vi "MAG_UI_Main.vi"() -> ()   [LabVIEW 2016]
doc: "Use this template to build a simple state machine design pattern. Each state executes code and determines which state to transition to."
uses:
  controls/MAG_UI_Data.ctl
  controls/MAG_UI_Command.ctl
  controls/MAG_Comms_State.ctl
  controls/Sensor_Data.ctl
  <vilib>/Math Plots/3D Math Plots/3D Surface/3D Surface XCtrl/3D Surface.xctl
  controls/MAG_UI_State.ctl
  controls/MAG_Display_State.ctl
  controls/MAG_UI_Comms_Config.ctl
  <vilib>/Math Plots/3D Math Plots/3D Surface/3D Surface Datatype/Public/Plot Helper (Matrix).vi
  <vilib>/Math Plots/3D Math Plots/3D Surface/3D Surface Datatype/3D Surface Datatype.lvclass
panel:
  in  "UI_Tab":enum32{"Display", "Config", "Debug"}(tab)
  out "Sensor Readings":dbl[][](array[numeric])=[[-533.0, -111.0, 239.0], [-402.0, 166.0, 184.0], [-184.0, 154.0, 29.0], [-106.0, 74.0, 11.0], [-532.0, -109.0, 246.0], [-398.0, 164.0, 175.0], [-205.0, 152.0, 32.0], [-119.0, 65.0, 9.0], [-529.0, -110.0, 242.0], [-408.0, 166.0, 184.0], [-198.0, 158.0, 27.0], [-108.0, 61.0, 6.0], [-539.0, -106.0, 240.0], [-407.0, 158.0, 183.0], [-191.0, 156.0, 28.0], [-113.0, 73.0, 15.0], [816.0, -260.0, 842.0], [539.0, 512.0, 512.0], [156.0, 425.0, 83.0], [13.0, 142.0, -72.0], [816.0, -262.0, 840.0], [528.0, 520.0, 512.0], [162.0, 425.0, 83.0], [13.0, 137.0, -84.0], [809.0, -260.0, 840.0], [538.0, 520.0, 504.0], [162.0, 432.0, 72.0], [13.0, 136.0, -84.0], [809.0, -260.0, 846.0], [538.0, 508.0, 512.0], [158.0, 435.0, 72.0], [19.0, 136.0, -79.0], [346.0, -168.0, 14.0], [287.0, -68.0, 19.0], [161.0, -34.0, 4.0], [70.0, -44.0, -7.0], [345.0, -191.0, 19.0], [279.0, -40.0, 8.0], [167.0, -16.0, 12.0], [72.0, -23.0, 2.0], [341.0, -190.0, 17.0], [285.0, -46.0, 9.0], [149.0, -15.0, 6.0], [54.0, -40.0, -2.0], [375.0, -201.0, 19.0], [282.0, -51.0, 10.0], [135.0, -37.0, 6.0], [81.0, -57.0, -12.0], [-80.0, -193.0, -48.0], [-73.0, -136.0, -12.0], [-5.0, -122.0, -31.0], [-19.0, -118.0, -17.0], [-118.0, -187.0, -48.0], [-73.0, -115.0, -22.0], [1.0, -113.0, -27.0], [-20.0, -111.0, -8.0], [-99.0, -184.0, -40.0], [-62.0, -145.0, -17.0], [0.0, -113.0, -37.0], [-7.0, -117.0, -15.0], [-126.0, -184.0, -50.0], [-72.0, -115.0, -14.0], [-4.0, -114.0, -25.0], [-29.0, -116.0, -14.0]]
  in  "Zero":bool=TRUE
  in  "Tab Control":enum32{"2D", "3D"}(tab)
  out "Node Response":T1(graph)
  in  "Node":i32
  out "3D Surface":refnum<class "3D Plot Datatype.lvclass">[](xcontrol)
  in  "Comms Setting":enum32{"Serial", "Bluetooth"}(tab)
  in  "VISA resource name":refnum<visa-resource-name>="COM11"
  in  "Serial Settings":T2={"baud rate"=115200, "data bits"=8, "parity"=enum."None", "stop bits"=10, "flow control"=0} {"flow control" items=["None"=0, "XON/XOFF"=1, "RTS/CTS"=2, "DTR/DSR"=4]; "stop bits" items=["1.0"=10, "1.5"=15, "2.0"=20]; "data bits" min=5 max=8 step=1; "baud rate" items=["75"=75, "110"=110, "134"=134, "150"=150, "300"=300, "600"=600, "1200"=1200, "1800"=1800, "2400"=2400, "4800"=4800, "7200"=7200, "9600"=9600, "14400"=14400, "19200"=19200, "28800"=28800, "38400"=38400, "56000"=56000, "57600"=57600, "115200"=115200, "128000"=128000, "230400"=230400]}
  out "Comm State":T3={"Comms_States"=enum."Send_Com", "Parameters"="", "Clear Buffer?"=FALSE}
  out "notification":T5
  out "comms":i32
  out "ui":i32
  in  "Button_Disconnect":bool
  in  "Button_Initialise":bool
  in  "Button_Stream":bool
  out "Status":T6
  in  "Button_Record":bool
  in  "Button_Sys_Check":bool
  in  "Button_Connect":bool
  in  "Button_Exit":bool
  # "MagBoard n64"
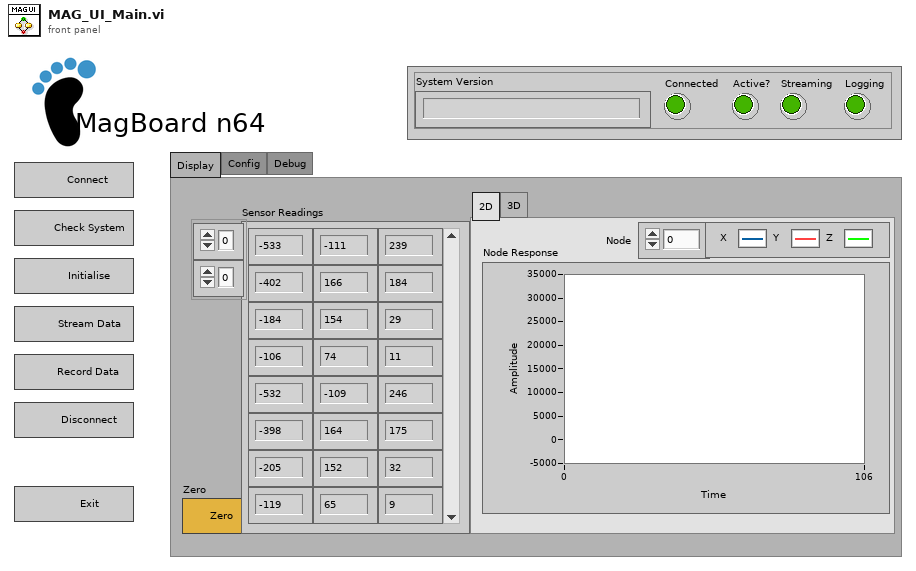
[diagram p1: front panel]
types:
  T1 = cluster{"Node XYZ List[0]":dbl, "Node XYZ List[1]":dbl, "Node XYZ List[2]":dbl}
  T2 = cluster{"baud rate":u32, "data bits":u16, "parity":enum16{"None", "Odd", "Even", "Mark", "Space"}, "stop bits":u16, "flow control":u16}
  T3 = typedef "MAG_UI_Command.ctl" = cluster{"Comms_States":T4, "Parameters":string, "Clear Buffer?":bool}
  T4 = typedef "MAG_Comms_State.ctl" = enum16{"Initialize", "Wait for Event", "Connect", "Send_Com", "Rcv_TXT", "Rcv_BIN", "Rcv_FILE", "Disconnect"}
  T5 = typedef "Sensor_Data.ctl" = cluster{"Time":u32, "Data":i16[]}
  T6 = typedef "MAG_UI_Data.ctl" = cluster{"System Version":string, "Connected":bool, "Active?":bool, "Streaming":bool, "Logging":bool}
  T7 = typedef "MAG_UI_Comms_Config.ctl" = cluster{enum16{"Serial", "Bluetooth"}, "Serial Refnum":refnum<visa-resource-name>}
  T8 = typedef "MAG_Display_State.ctl" = enum16{"Initialise", "Display", "Exit"}
  T9 = typedef "MAG_UI_State.ctl" = enum16{"Initialize", "Wait for Event", "Com_Connect", "Com_Init_Sys", "Com_Chk_Sys", "Com_Stream", "Com_Log", "Exit"}
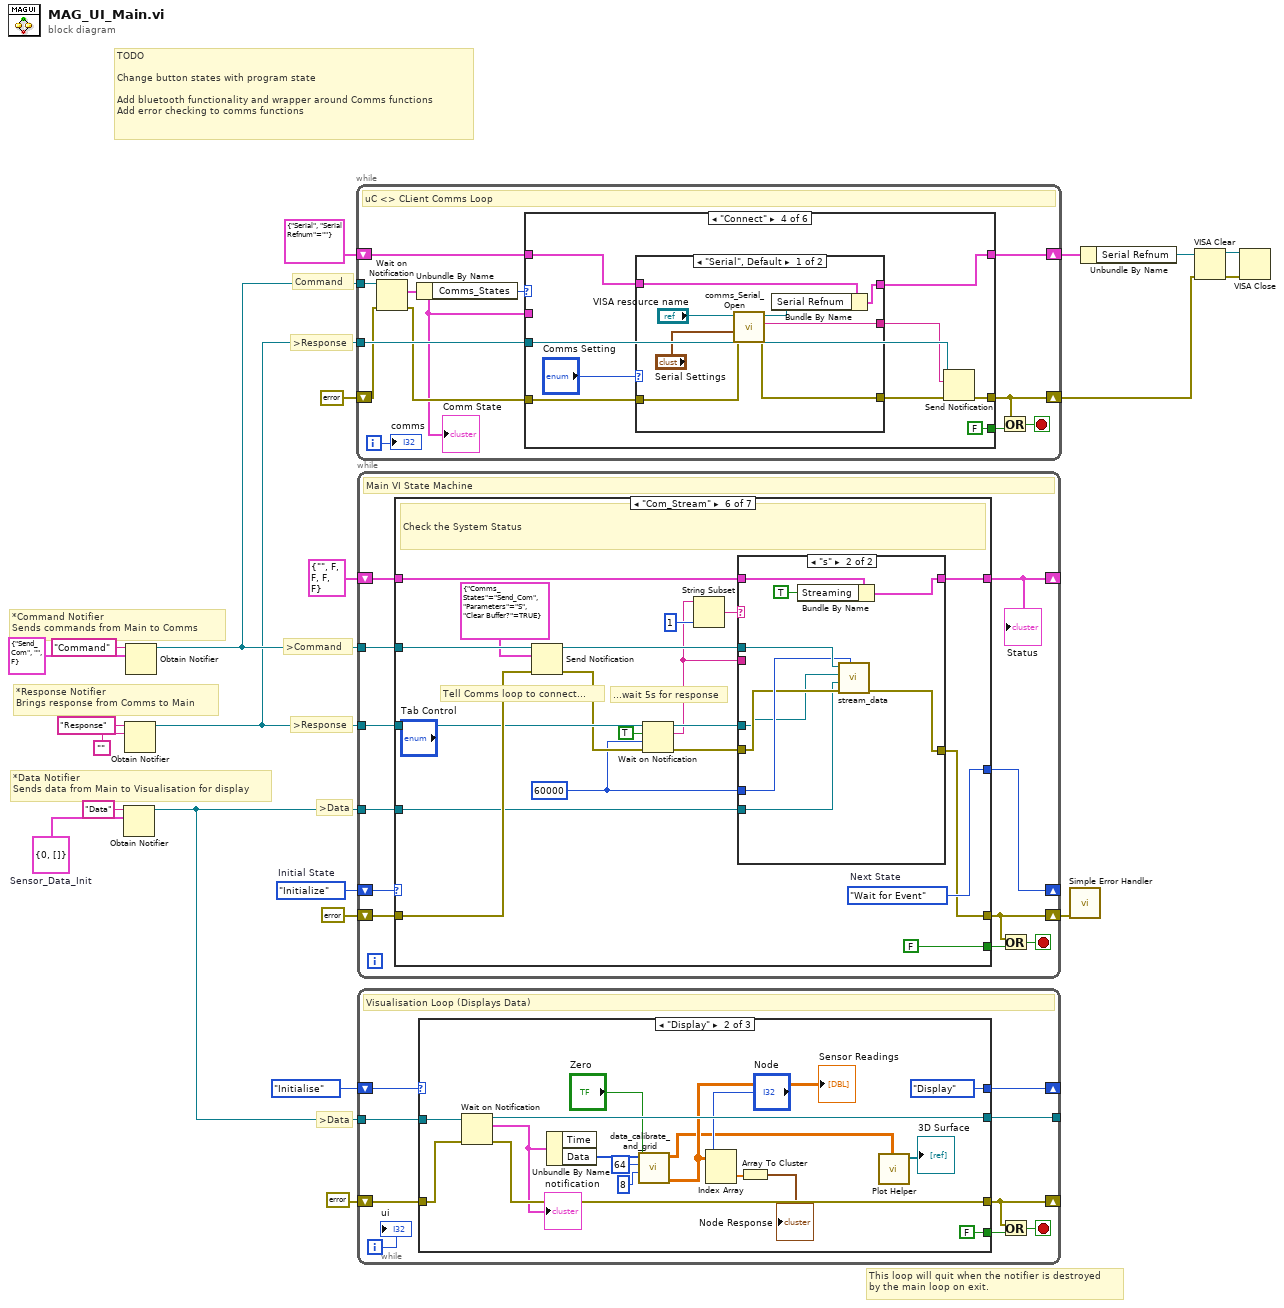
[diagram p0: block diagram]
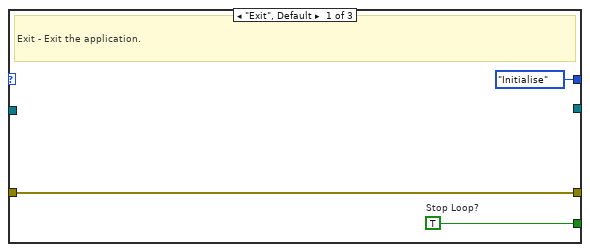
[diagram p2: hidden frame]
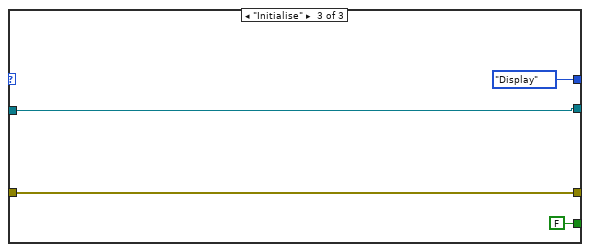
[diagram p3: hidden frame]
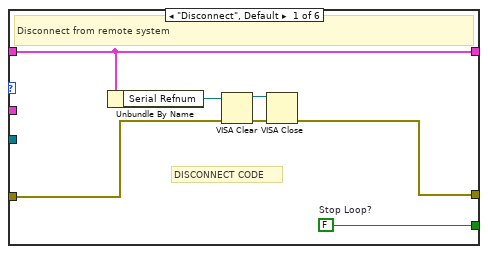
[diagram p4: hidden frame]
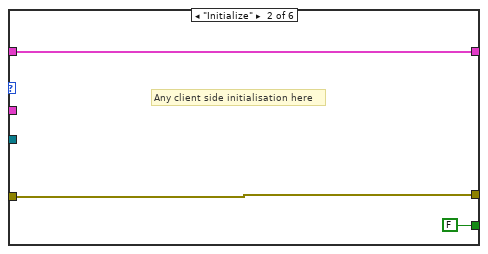
[diagram p5: hidden frame]
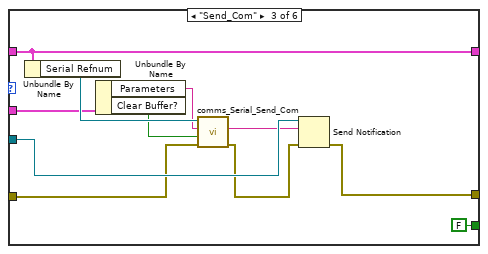
[diagram p6: hidden frame]
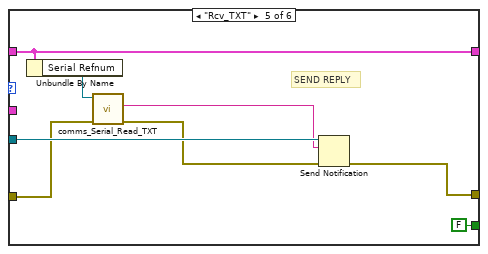
[diagram p8: hidden frame]
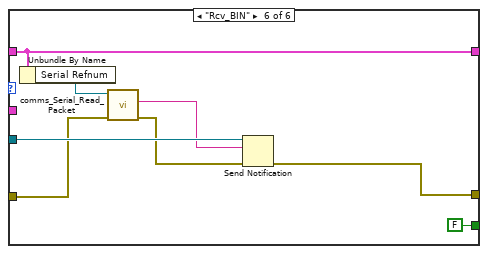
[diagram p9: hidden frame]
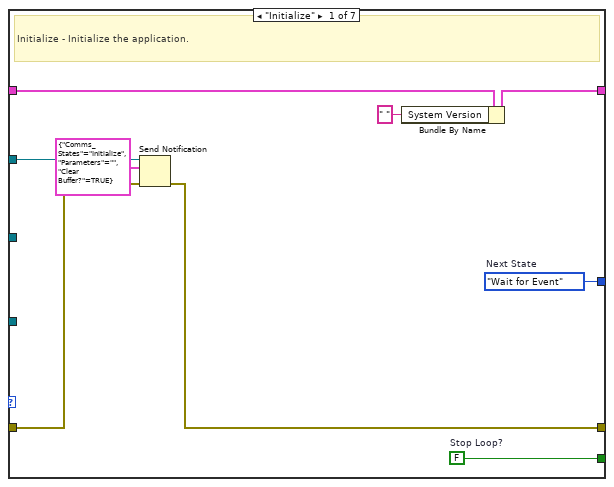
[diagram p10: hidden frame]
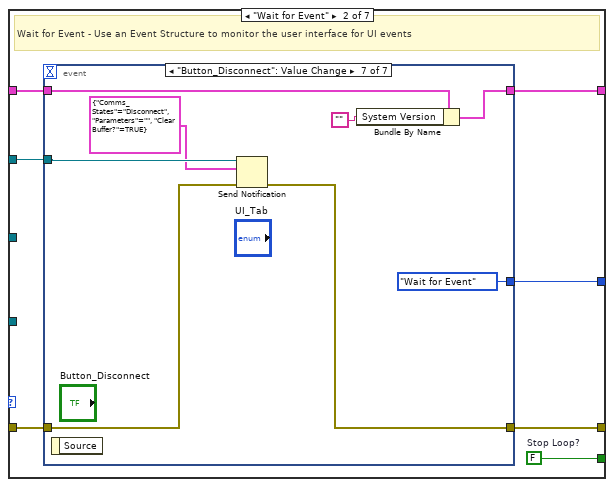
[diagram p11: hidden frame]
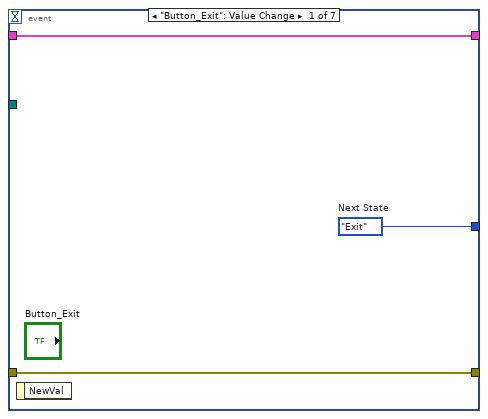
[diagram p12: hidden frame]
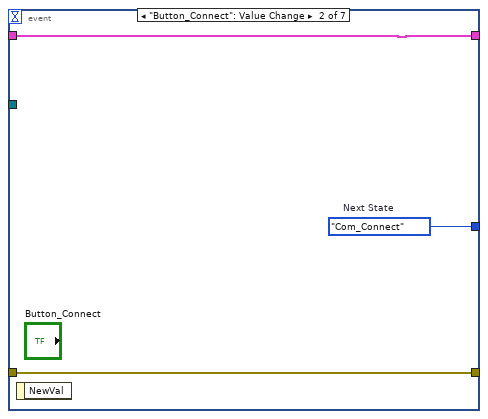
[diagram p13: hidden frame]
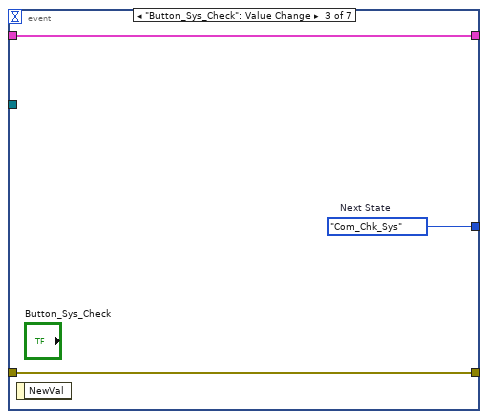
[diagram p14: hidden frame]
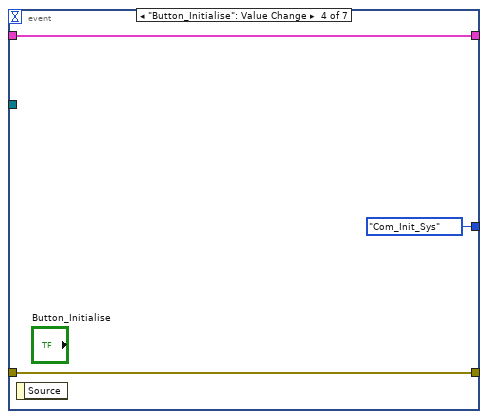
[diagram p15: hidden frame]
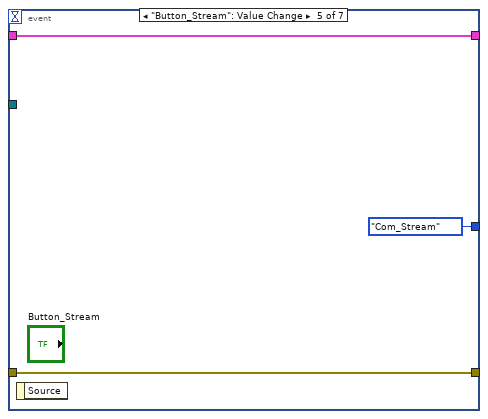
[diagram p16: hidden frame]
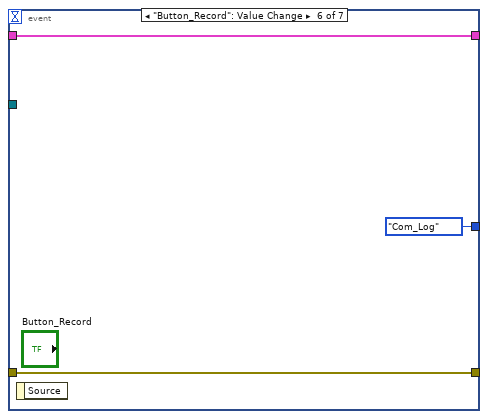
[diagram p17: hidden frame]
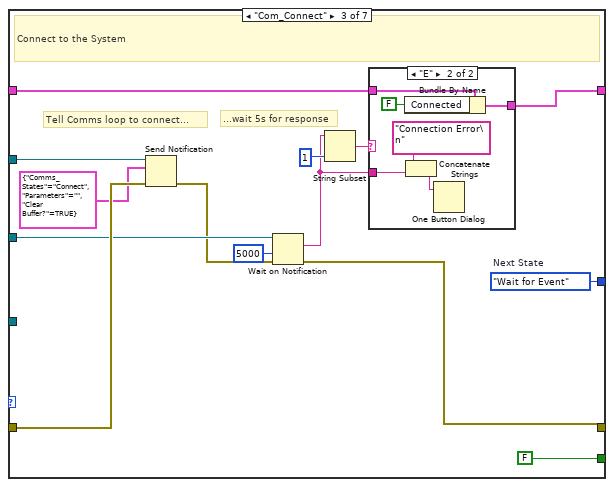
[diagram p18: hidden frame]
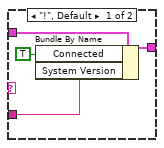
[diagram p19: hidden frame]
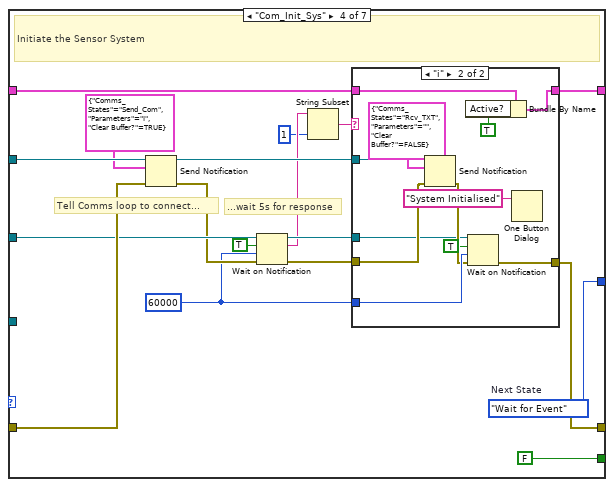
[diagram p20: hidden frame]
diagram:
  w10 = T5 {"Time"=0, "Data"=[]}  # Sensor_Data_Init
  w22 = MAG_UI_State."Initialize"  # Initial State
  # "TODO\n\nChange button states with program state\n\nAdd bluetooth functionality and wrapper around Comms functions\nAdd error checking to comms functions"
  # "This loop will quit when the notifier is destroyed\nby the main loop on exit."
  # ">Data"
  # ">Data"
  # ">Response"
  # ">Response"
  # ">Command"
  # "*Data Notifier\nSends data from Main to Visualisation for display"
  # "*Response Notifier\nBrings response from Comms to Main"
  # "*Command Notifier\nSends commands from Main to Comms"
  # "Command"
  n1 = Obtain Notifier(name (unnamed)="Data", notification data type=w10) -> (notifier out=w13:refnum<notifier>)  [unwired: 2 in, 2 out]
  n2 = Obtain Notifier(name (unnamed)="Response", notification data type="") -> (notifier out=w12:refnum<notifier>)  [unwired: 2 in, 2 out]
  n3 = Obtain Notifier(name (unnamed)="Command", notification data type=T3 {"Comms_States"=enum."Send_Com", "Parameters"="", "Clear Buffer?"=FALSE}) -> (notifier out=w16:refnum<notifier>)  [unwired: 2 in, 2 out]
  n4 = while {
    shift-right: [w31] -> w1
    shift-left: errorcluster {"status"=FALSE, "code"=0, "source"=""} ("error constant") -> [w28]
    tunnel: w16 -> [w30]
    tunnel: w12 -> [w32]
    shift-right: [w25] -> w2
    shift-left: T7 {enum."Serial", "Serial Refnum"=""} -> [w26]
    i -> [w24]
    stop <- w33 stop-if-true
    # "uC <> CLient Comms Loop"
    n5 = Wait on Notification(notifier=w30, error in (no error)=w28) -> (notification=w23:T3, error out=w27:errorcluster)  [unwired: 2 in, 2 out]
    "Comm State" <- w23
    n6 = Unbundle By Name(w23) -> ("Comms_States"=w29:T4)
    n7 = case shown="\"Connect\"" w29 {
      tunnel: [w41 FALSE ("Stop Loop?") FALSE ("Stop Loop?") FALSE ("Stop Loop?") FALSE ("Stop Loop?") FALSE ("Stop Loop?")] -> w34
      tunnel: w27 -> [w37 w43 w49 w57 w77 w84]
      tunnel: [w36 w43 w54 w64 w81 w89] -> w31
      tunnel: w32 -> [_ _ w55 w61 w82 w88]
      tunnel: w26 -> [w35 w42 w50 w59 w79 w85]
      tunnel: [w35 w42 w50 w58 w79 w85] -> w25
      tunnel: w23 -> [_ _ w46 _ _ _]
      frame "Disconnect", Default {
        w41 = FALSE  # Stop Loop?
        # "DISCONNECT CODE"
        # "Disconnect from remote system"
        n8 = Unbundle By Name(w35) -> ("Serial Refnum"=w40:refnum<visa-resource-name>)
        n9 = VISA Clear(VISA resource name=w40, error in (no error)=w37) -> (VISA resource name out=w38:refnum<visa-resource-name>, error out=w39:errorcluster)
        n10 = VISA Close(VISA resource name=w38, error in (no error)=w39) -> (error out=w36:errorcluster)
      }
      frame "Initialize" {
        # "Any client side initialisation here"
      }
      frame "Send_Com" {
        n11 = Unbundle By Name(w50) -> ("Serial Refnum"=w52:refnum<visa-resource-name>)
        n12 = Unbundle By Name(w46) -> ("Parameters"=w45:string, "Clear Buffer?"=w47:bool)
        n13 = call "comms_Serial_Send_Com.vi"("error in"=w49, "Buffer Clear?"=w47, "Command"=w45, "VISA resource in"=w52) -> ("error out"=w48:errorcluster, "Response"=w51:string)  [unwired: 5 in, 1 out]
        n14 = Send Notification(notification=w51, notifier=w55, error in (no error)=w48) -> (error out=w54:errorcluster)  [unwired: 1 out]
      }
      frame "Connect" {
        n15 = case shown="\"Serial\", Default" "Comms Setting" {
          tunnel: [w66 w73] -> w60
          tunnel: w59 -> [w70 w74]
          tunnel: [w68 w74] -> w58
          tunnel: w57 -> [w67 w73]
          tunnel: [w65 _] -> w56
          frame "Serial", Default {
            n16 = call "comms_Serial_Open.vi"("error in (no error)"=w67, "Serial Settings in"="Serial Settings", "VISA Refnum in"="VISA resource name") -> ("error out"=w66:errorcluster, "Data Out"=w65:string, "VISA Refnum out"=w69:refnum<visa-resource-name>)  [unwired: 6 in]
            n17 = Bundle By Name(cluster=w70, "Serial Refnum"=w69) -> (w68:T7)
          }
          frame "Bluetooth" {
          }
        }
        n18 = Send Notification(notification=w56, notifier=w61, error in (no error)=w60) -> (error out=w64:errorcluster)  [unwired: 1 out]
      }
      frame "Rcv_TXT" {
        # "SEND REPLY"
        n19 = Unbundle By Name(w79) -> ("Serial Refnum"=w78:refnum<visa-resource-name>)
        n20 = call "comms_Serial_Read_TXT.vi"("error in"=w77, "VISA resource in"=w78) -> ("error out"=w76:errorcluster, "Data Out"=w75:string)  [unwired: 6 in, 2 out]
        n21 = Send Notification(notification=w75, notifier=w82, error in (no error)=w76) -> (error out=w81:errorcluster)  [unwired: 1 out]
      }
      frame "Rcv_BIN" {
        n22 = Unbundle By Name(w85) -> ("Serial Refnum"=w86:refnum<visa-resource-name>)
        n23 = call "comms_Serial_Read_Packet.vi"("error in"=w84, "VISA resource in"=w86) -> ("error out"=w83:errorcluster, "Data Out"=w87:string)  [unwired: 7 in, 1 out]
        n24 = Send Notification(notification=w87, notifier=w88, error in (no error)=w83) -> (error out=w89:errorcluster)  [unwired: 1 out]
      }
    }
    n25 = Or(x=w31, y=w34) -> (x .or. y?=w33:bool)
    "comms" <- w24
  }
  n26 = while {
    shift-right: [w100] -> _
    shift-left: w22 -> [w101]
    shift-right: [w91] -> _
    shift-left: T6 {"System Version"="", "Connected"=FALSE, "Active?"=FALSE, "Streaming"=FALSE, "Logging"=FALSE} ("Data") -> [w99]
    shift-right: [w95] -> w19
    shift-left: errorcluster {"status"=FALSE, "code"=0, "source"=""} ("error constant") -> [w98]
    tunnel: w16 -> [w94]
    tunnel: w12 -> [w93]
    tunnel: w13 -> [w92]
    stop <- w96 stop-if-true
    # "Main VI State Machine"
    n27 = case shown="\"Com_Stream\"" w101 {
      tunnel: [w110 w117 w157 w176 w213 w249 w285] -> w100
      tunnel: [w109 w116 FALSE ("Stop Loop?") FALSE ("Stop Loop?") FALSE ("Stop Loop?") FALSE ("Stop Loop?") w283] -> w97
      tunnel: w99 -> [w108 w115 w149 w180 w217 w253 w284]
      tunnel: [w107 w114 w148 w179 w216 w252 w284] -> w91
      tunnel: w98 -> [w103 w113 w154 w183 w220 w256 w279]
      tunnel: [w102 w112 w151 w173 w210 w246 w278] -> w95
      tunnel: w94 -> [w105 w111 w155 w184 w221 w257 w282]
      tunnel: w93 -> [_ _ w153 w182 w219 w255 w276]
      tunnel: w92 -> [_ _ _ _ _ w242 w275]
      frame "Initialize" {
        w109 = FALSE  # Stop Loop?
        w110 = MAG_UI_State."Wait for Event"  # Next State
        # "Initialize - Initialize the application."
        n28 = Send Notification(notification=T3 {"Comms_States"=enum."Initialize", "Parameters"="", "Clear Buffer?"=TRUE}, notifier=w105, error in (no error)=w103) -> (error out=w102:errorcluster)  [unwired: 1 out]
        n29 = Bundle By Name(cluster=w108, "System Version"=" ") -> (w107:T6)
      }
      frame "Wait for Event" {
        w116 = FALSE  # Stop Loop?
        # "Wait for Event - Use an Event Structure to monitor the user interface for UI events"
        n30 = event shown="[6] \"Button_Disconnect\": Value Change" {
          selector: _ -> [_ _ _ _ _ _ _]
          dyn-events: _ -> [_ _ _ _ _ _ _]
          timeout: _ -> [_ _ _ _ _ _ _]
          tunnel: [w120 w123 w126 MAG_UI_State."Com_Init_Sys" ("Next State") MAG_UI_State."Com_Stream" ("Next State") MAG_UI_State."Com_Log" ("Next State") MAG_UI_State."Wait for Event" ("Next State")] -> w117
          tunnel: w115 -> [w119 w121 w124 w129 w132 w135 w138]
          tunnel: [w119 w121 w124 w129 w132 w135 w137] -> w114
          tunnel: w113 -> [w118 w122 w125 w128 w131 w134 w141]
          tunnel: [w118 w122 w125 w128 w131 w134 w140] -> w112
          tunnel: w111 -> [_ _ _ _ _ _ w142]
          event "Button_Exit": Value Change {
            w120 = MAG_UI_State."Exit"  # Next State
            n31 = event-data() -> ()  [unwired: 1 in, 1 out]
          }
          event "Button_Connect": Value Change {
            w123 = MAG_UI_State."Com_Connect"  # Next State
            n32 = event-data() -> ()  [unwired: 1 in, 1 out]
          }
          event "Button_Sys_Check": Value Change {
            w126 = MAG_UI_State."Com_Chk_Sys"  # Next State
            n33 = event-data() -> ()  [unwired: 1 in, 1 out]
          }
          event "Button_Initialise": Value Change {
            n34 = event-data() -> ()  [unwired: 1 in, 1 out]
          }
          event "Button_Stream": Value Change {
            n35 = event-data() -> ()  [unwired: 1 in, 1 out]
          }
          event "Button_Record": Value Change {
            n36 = event-data() -> ()  [unwired: 1 in, 1 out]
          }
          event "Button_Disconnect": Value Change {
            n37 = event-data() -> ()  [unwired: 1 in, 1 out]
            n38 = Send Notification(notification=T3 {"Comms_States"=enum."Disconnect", "Parameters"="", "Clear Buffer?"=TRUE}, notifier=w142, error in (no error)=w141) -> (error out=w140:errorcluster)  [unwired: 1 out]
            n39 = Bundle By Name(cluster=w138, "System Version"="") -> (w137:T6)
          }
        }
      }
      frame "Com_Connect" {
        w157 = MAG_UI_State."Wait for Event"  # Next State
        # "...wait 5s for response"
        # "Tell Comms loop to connect..."
        # "Connect to the System"
        n40 = Send Notification(notification=T3 {"Comms_States"=enum."Connect", "Parameters"="", "Clear Buffer?"=TRUE}, notifier=w155, error in (no error)=w154) -> (error out=w152:errorcluster)  [unwired: 1 out]
        n41 = Wait on Notification(notifier=w153, timeout in ms (-1)=5000, error in (no error)=w152) -> (notification=w144:string, error out=w151:errorcluster)  [unwired: 1 in, 2 out]
        n42 = String Subset(string=w144, length (rest)=1 ("offset (0)")) -> (substring=w146:string)  [unwired: 1 in]
        n43 = case shown="\"E\"" w146 {
          tunnel: w149 -> [w161 w165]
          tunnel: [w160 w164] -> w148
          tunnel: w144 -> [w158 w162]
          frame "!", Default {
            n44 = Bundle By Name(cluster=w161, "Connected"=TRUE, "System Version"=w158) -> (w160:T6)
          }
          frame "E" {
            n45 = Bundle By Name(cluster=w165, "Connected"=FALSE) -> (w164:T6)
            n46 = Concatenate Strings("Connection Error\n", w162) -> (w167:string)
            n47 = One Button Dialog(message=w167) -> ()  [unwired: 1 in, 1 out]
          }
        }
      }
      frame "Com_Init_Sys" {
        w176 = MAG_UI_State."Wait for Event"  # Next State
        w175 = 60000 ("timeout in ms (-1)")
        # "...wait 5s for response"
        # "Tell Comms loop to connect..."
        # "Initiate the Sensor System"
        n48 = Send Notification(notification=T3 {"Comms_States"=enum."Send_Com", "Parameters"="I", "Clear Buffer?"=TRUE}, notifier=w184, error in (no error)=w183) -> (notifier out=w177:refnum<notifier>, error out=w181:errorcluster)
        n49 = Wait on Notification(notifier=w182, ignore previous (F)=TRUE, timeout in ms (-1)=w175, error in (no error)=w181) -> (notifier out=w172:refnum<notifier>, notification=w169:string, error out=w174:errorcluster)  [unwired: 1 out]
        n50 = String Subset(string=w169, length (rest)=1 ("offset (0)")) -> (substring=w170:string)  [unwired: 1 in]
        n51 = case shown="\"i\"" w170 {
          selector: w170 -> [w190 _]
          tunnel: w180 -> [w189 w196]
          tunnel: [w188 w195] -> w179
          tunnel: w177 -> [_ w203]
          tunnel: w175 -> [_ w202]
          tunnel: w174 -> [w186 w201]
          tunnel: [w186 w199] -> w173
          tunnel: w172 -> [_ w198]
          frame "E", Default {
            n52 = Bundle By Name(cluster=w189, "Connected"=FALSE) -> (w188:T6)
            n53 = Concatenate Strings("Initialisation Failed", w190) -> (w192:string)
            n54 = One Button Dialog(message=w192) -> ()  [unwired: 1 in, 1 out]
          }
          frame "i" {
            n55 = Send Notification(notification=T3 {"Comms_States"=enum."Rcv_TXT", "Parameters"="", "Clear Buffer?"=FALSE}, notifier=w203, error in (no error)=w201) -> (error out=w200:errorcluster)  [unwired: 1 out]
            n56 = Bundle By Name(cluster=w196, "Active?"=TRUE) -> (w195:T6)
            n57 = Wait on Notification(notifier=w198, ignore previous (F)=TRUE, timeout in ms (-1)=w202, error in (no error)=w200) -> (error out=w199:errorcluster)  [unwired: 3 out]
            n58 = One Button Dialog(message="System Initialised") -> ()  [unwired: 1 in, 1 out]
          }
        }
      }
      frame "Com_Chk_Sys" {
        w213 = MAG_UI_State."Wait for Event"  # Next State
        w212 = 5000 ("timeout in ms (-1)")
        # "...wait 5s for response"
        # "Tell Comms loop to connect..."
        # "Check the System Status"
        n59 = Send Notification(notification=T3 {"Comms_States"=enum."Send_Com", "Parameters"="C", "Clear Buffer?"=TRUE}, notifier=w221, error in (no error)=w220) -> (notifier out=w214:refnum<notifier>, error out=w218:errorcluster)
        n60 = Wait on Notification(notifier=w219, ignore previous (F)=TRUE, timeout in ms (-1)=w212, error in (no error)=w218) -> (notifier out=w209:refnum<notifier>, notification=w206:string, error out=w211:errorcluster)  [unwired: 1 out]
        n61 = String Subset(string=w206, length (rest)=1 ("offset (0)")) -> (substring=w207:string)  [unwired: 1 in]
        n62 = case shown="\"c\"" w207 {
          selector: w207 -> [w227 _]
          tunnel: w217 -> [w226 w239]
          tunnel: [w225 w239] -> w216
          tunnel: w214 -> [_ w237]
          tunnel: w212 -> [_ w236]
          tunnel: w211 -> [w223 w235]
          tunnel: [w223 w233] -> w210
          tunnel: w209 -> [_ w232]
          frame "E", Default {
            n63 = Bundle By Name(cluster=w226, "Connected"=FALSE) -> (w225:T6)
            n64 = Concatenate Strings("Initialisation Failed", w227) -> (w229:string)
            n65 = One Button Dialog(message=w229) -> ()  [unwired: 1 in, 1 out]
          }
          frame "c" {
            n66 = Send Notification(notification=T3 {"Comms_States"=enum."Rcv_TXT", "Parameters"="", "Clear Buffer?"=FALSE}, notifier=w237, error in (no error)=w235) -> (error out=w234:errorcluster)  [unwired: 1 out]
            n67 = Wait on Notification(notifier=w232, ignore previous (F)=TRUE, timeout in ms (-1)=w236, error in (no error)=w234) -> (notification=w231:string, error out=w233:errorcluster)  [unwired: 2 out]
            n68 = One Button Dialog(message=w231) -> ()  [unwired: 1 in, 1 out]
          }
        }
      }
      frame "Com_Stream" {
        w249 = MAG_UI_State."Wait for Event"  # Next State
        w248 = 60000 ("timeout in ms (-1)")
        # "...wait 5s for response"
        # "Tell Comms loop to connect..."
        # "Check the System Status"
        n69 = Send Notification(notification=T3 {"Comms_States"=enum."Send_Com", "Parameters"="S", "Clear Buffer?"=TRUE}, notifier=w257, error in (no error)=w256) -> (notifier out=w250:refnum<notifier>, error out=w254:errorcluster)
        n70 = Wait on Notification(notifier=w255, ignore previous (F)=TRUE, timeout in ms (-1)=w248, error in (no error)=w254) -> (notifier out=w245:refnum<notifier>, notification=w240:string, error out=w247:errorcluster)  [unwired: 1 out]
        n71 = String Subset(string=w240, length (rest)=1 ("offset (0)")) -> (substring=w243:string)  [unwired: 1 in]
        n72 = case shown="\"s\"" w243 {
          tunnel: w253 -> [w263 w268]
          tunnel: [w262 w266] -> w252
          tunnel: w250 -> [_ w274]
          tunnel: w248 -> [_ w273]
          tunnel: w247 -> [w260 w272]
          tunnel: [w260 w271] -> w246
          tunnel: w245 -> [_ w270]
          tunnel: w242 -> [_ w269]
          tunnel: w240 -> [w259 _]
          frame "E", Default {
            n73 = Bundle By Name(cluster=w263, "Connected"=FALSE) -> (w262:T6)
            n74 = Concatenate Strings("Stream Failed", w259) -> (w265:string)
            n75 = One Button Dialog(message=w265) -> ()  [unwired: 1 in, 1 out]
          }
          frame "s" {
            n76 = Bundle By Name(cluster=w268, "Streaming"=TRUE) -> (w266:T6)
            n77 = call "stream_data.vi"("timeout in ms (-1)"=w273, "error in (no error)"=w272, "Display"=w269, "Response"=w270, "Command"=w274) -> ("error out"=w271:errorcluster)  [unwired: 6 in]
          }
        }
      }
      frame "Exit", Default {
        w277 = FALSE ("force destroy? (F)")
        w283 = TRUE  # Stop Loop?
        w285 = MAG_UI_State."Exit"  # (Value Not Used)
        # "Exit - Exit the application."
        n78 = Release Notifier(notifier=w282, force destroy? (F)=w277, error in (no error)=w279) -> (error out=w281:errorcluster)  [unwired: 2 out]
        n79 = Release Notifier(notifier=w276, force destroy? (F)=w277, error in (no error)=w281) -> (error out=w280:errorcluster)  [unwired: 2 out]
        n80 = Release Notifier(notifier=w275, force destroy? (F)=w277, error in (no error)=w280) -> (error out=w278:errorcluster)  [unwired: 2 out]
      }
    }
    "Status" <- w91
    n81 = Or(x=w95, y=w97) -> (x .or. y?=w96:bool)
  }
  n82 = while {
    shift-right: [w293] -> _
    shift-left: MAG_Display_State."Initialise" -> [w294]
    shift-right: [w289] -> _
    shift-left: errorcluster {"status"=FALSE, "code"=0, "source"=""} ("error constant") -> [w292]
    tunnel: w13 -> [w288]
    tunnel: [w287] -> _
    i -> [w286]
    stop <- w290 stop-if-true
    # "Visualisation Loop (Displays Data)"
    n83 = case shown="\"Display\"" w294 {
      tunnel: [MAG_Display_State."Initialise" MAG_Display_State."Display" MAG_Display_State."Display"] -> w293
      tunnel: [w297 FALSE ("Stop Loop?") FALSE ("Stop Loop?")] -> w291
      tunnel: w292 -> [w296 w311 w318]
      tunnel: [w296 w310 w318] -> w289
      tunnel: w288 -> [_ w312 w315]
      tunnel: [_ w309 w315] -> w287
      frame "Exit", Default {
        w297 = TRUE  # Stop Loop?
        # "Exit - Exit the application."
      }
      frame "Display" {
        n84 = Wait on Notification(notifier=w312, error in (no error)=w311) -> (notifier out=w309:refnum<notifier>, notification=w306:T5, error out=w310:errorcluster)  [unwired: 2 in, 1 out]
        "notification" <- w306
        n85 = Unbundle By Name(w306) -> ("Data"=w305:i16[])  [unwired: 1 out]
        n86 = call "data_calibrate_and_grid.vi"("Tare"="Zero", "Row Length"=8, "No. Nodes"=64, "Sensor Readings (PACKET)"=w305) -> ("Node XYZ List"=w301:dbl[][], "Z (GRID)"=w298:dbl[][])  [unwired: 3 in, 3 out]
        "Sensor Readings" <- w301
        n87 = Index Array(array=w301, index (row)="Node") -> (element=w308:dbl[])  [unwired: 1 in]
        n88 = Array To Cluster(array=w308) -> (cluster=→"Node Response":T1)
        n89 = call-poly <vilib>:"Plot Helper.vi"("z matrix"=w298) -> ("3D Plot lvclass Array out"=→"3D Surface":refnum<class "3D Plot Datatype.lvclass">[])  [unwired: 5 in, 5 out]
      }
      frame "Initialise" {
      }
    }
    n90 = Or(x=w289, y=w291) -> (x .or. y?=w290:bool)
    "ui" <- w286
  }
  n91 = call <vilib>:"Simple Error Handler.vi"("error in (no error)"=w19) -> ()  [unwired: 4 in, 5 out]
  n92 = Unbundle By Name(w2) -> ("Serial Refnum"=w3:refnum<visa-resource-name>)
  n93 = VISA Clear(VISA resource name=w3, error in (no error)=w1) -> (VISA resource name out=w5:refnum<visa-resource-name>, error out=w4:errorcluster)
  n94 = VISA Close(VISA resource name=w5, error in (no error)=w4) -> ()  [unwired: 1 out]
